vi "CMN_number2binarystr.vi"(10 "decimal number":u32) -> (1 "Numeric":u32 format="%.0b", 2 "binary string":string)   [LabVIEW 2016]
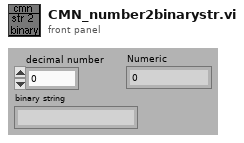
[diagram p1: front panel]
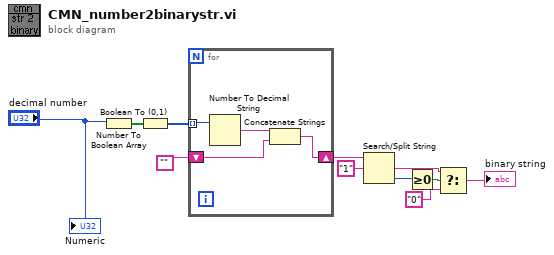
[diagram p0: block diagram]
diagram:
  n1 = Number To Boolean Array(number="decimal number") -> (Boolean array=w10:bool[])
  n2 = Boolean To (0,1)(Boolean=w10) -> (0, 1=w9:i16[])
  n3 = for {
    tunnel: w9 -> [w15] mode=indexing
    shift-right: [w13] -> w7
    shift-left: "" -> [w12]
    n4 = Number To Decimal String(number=w15) -> (decimal integer string=w14:string)  [unwired: 1 out]
    n5 = Concatenate Strings(w14, w12) -> (w13:string)
  }
  n6 = Search/Split String(string=w7, search string/char (-)="1") -> (match + rest of string=w3:string, offset of match=w5:i32)  [unwired: 2 out]
  n7 = Greater Or Equal To 0?(x=w5) -> (x >= 0?=w4:bool)
  n8 = Select(t=w3, s=w4, f="0") -> (s? t:f=→"binary string":string)
  "Numeric" <- "decimal number"
